vi "Create Zero Padded String.vi"(5 "Width":i32, 9 "Value":u32) -> (8 "Zero Padded Value":string)   [LabVIEW 2016]
doc: "Applies a prefix of 0's such that the output string length is equal to the input <b>width</b>."
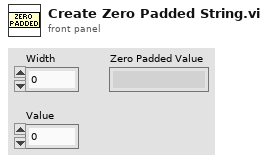
[diagram p1: front panel]
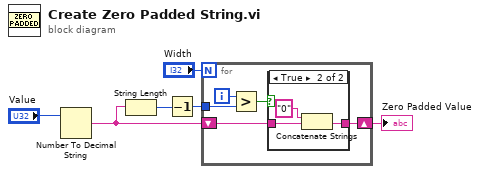
[diagram p0: block diagram]
diagram:
  n1 = Number To Decimal String(number="Value") -> (decimal integer string=w3:string)  [unwired: 1 in]
  n2 = String Length(string=w3) -> (length=w4:i32)
  n3 = Decrement(x=w4) -> (x-1=w5:i32)
  n4 = for {
    N: "Width" -> [_]
    shift-right: [w7] -> w6
    shift-left: w3 -> [w8]
    tunnel: w5 -> [w10]
    i -> [w11]
    n5 = Greater?(x=w11, y=w10) -> (0:w9:bool)
    n6 = case shown="True" w9 {
      tunnel: w8 -> [w12 w15]
      tunnel: [w12 w13] -> w7
      frame False {
      }
      frame True {
        n7 = Concatenate Strings("0" ("string"), w15) -> (w13:string)
      }
    }
  }
  "Zero Padded Value" <- w6
